vi "16-bit display mapping.vi"(8 "error in (no error)":errorcluster) -> (0 "error out":errorcluster)   [LabVIEW 2020]
uses:
  Globals/gl_Time series viewer globals.vi
panel:
  out "error out 2":errorcluster
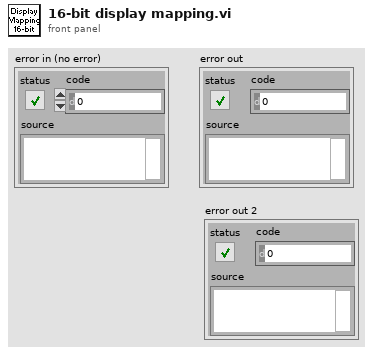
[diagram p1: front panel]
types:
  T1 = cluster{"Conversion Method":u32, "Minimum Value":i32, "Maximum Value":i32, "Number Of Shifts":i32}
  T2 = typedef "Time series viewer refs.ctl" = cluster{"This VI":refnum<vi>, "Image control":refnum<vi>, "AVI Mode ind":refnum<vi>, "Play":refnum<vi>, "Stop":refnum<vi>, "Back":refnum<vi>, "Scrollbar":refnum<vi>, "Video length info":refnum<vi>, "Expected speed values":refnum<vi>, "Intensity":refnum<vi>, "Path":refnum<vi>, "Selection sliders":refnum<vi>, "Speed Graph ref":refnum<vi>, "Frame rate set (fps)":refnum<vi>, "Number of rows to generate":refnum<vi>, "VL Image Array":refnum<vi>, "Image Scrollbar":refnum<vi>, "Channel to load":refnum<vi>, "Colour":refnum<vi>}
  T3 = typedef "Custom slider-horisontal.ctl" = cluster{dbl, dbl}
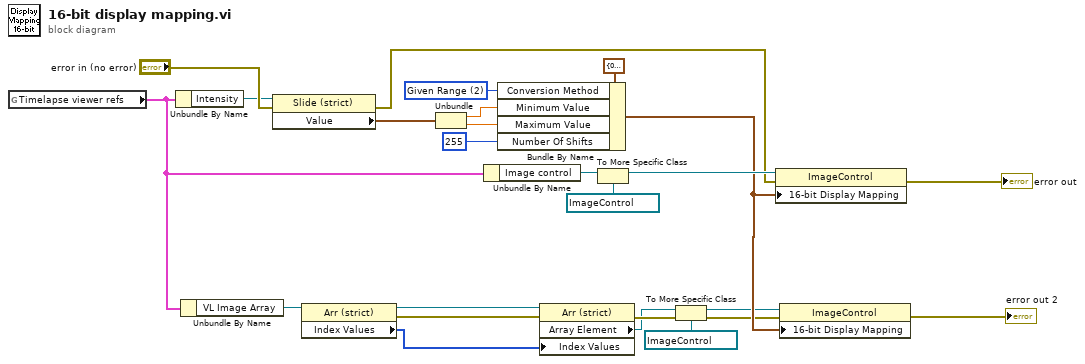
[diagram p0: block diagram]
diagram:
  w23 = u32 2 items=["Full Dynamic", "Downshift", "Given Range", "90% Dynamic", "Given Percent Range"] ("16-bit Display Mapping:Conversion Method")
  n1 = global read "gl_Time series viewer globals.vi" "Timelapse viewer refs"() -> (w12:T2)
  n2 = Unbundle By Name(w12) -> ("Intensity"=w18:refnum<vi>)
  n3 = Unbundle By Name(w12) -> ("VL Image Array"=w10:refnum<vi>)
  n4 = property on="Property Node" class="Slide (strict)"(reference=w18, error in="error in (no error)") -> (error out=w13:errorcluster, "Value"=w24:T3)  [unwired: 1 out]
  n5 = property class="Arr (strict)"(reference=w10) -> (reference out=w9:refnum<vi>, error out=w8:errorcluster, "Index Values"=w1:u32[])  [unwired: 1 in]
  n6 = Unbundle(w24) -> (w21:dbl, w22:dbl)
  n7 = Unbundle By Name(w12) -> ("Image control"=w16:refnum<vi>)
  n8 = Bundle By Name(cluster=T1 {"Conversion Method"=0, "Minimum Value"=0, "Maximum Value"=0, "Number Of Shifts"=0} ("16-bit Display Mapping:All Elements"), "Conversion Method"=w23, "Minimum Value"=w21, "Maximum Value"=w22, "Number Of Shifts"=255) -> (w11:T1)
  n9 = property class="Arr (strict)"(reference=w9, error in=w8, "Index Values"=w1) -> (error out=w4:errorcluster, "Array Element"=w2:refnum<vi>)  [unwired: 1 out]
  n10 = To More Specific Class(target class=refnum<vi> refnum ("Image"), reference=w16) -> (specific class reference=w15:refnum<vi>)  [unwired: 1 in, 1 out]
  n11 = To More Specific Class(target class=refnum<vi> refnum ("Image"), reference=w2, error in=w4) -> (specific class reference=w5:refnum<vi>, error out=w3:errorcluster)
  n12 = property on="Property Node" class="ImageControl"(reference=w15, error in=w13, "16-bit Display Mapping"=w11) -> (error out=→"error out":errorcluster)  [unwired: 1 out]
  n13 = property on="Property Node" class="ImageControl"(reference=w5, error in=w3, "16-bit Display Mapping"=w11) -> (error out=→"error out 2":errorcluster)  [unwired: 1 out]
